vi "Allan-Variance_Algorithm.VI"(1 "tau":dbl, 2 "Input Array":dbl[](array[numeric])) -> (0 "Allan-Varianz (tau)":dbl)   [LabVIEW 2020]
uses:
  <vilib>/Analysis/baseanly.llb/Mean (DBL).vi
  <vilib>/Analysis/NI_AALBase.lvlib
panel:
  out "[y_mean(k+1) - y_mean(k)]**2":dbl[](array[numeric]) format="%_3f"
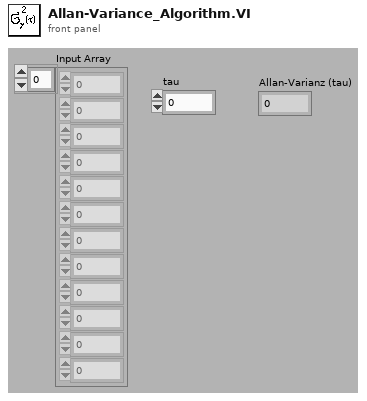
[diagram p1: front panel]
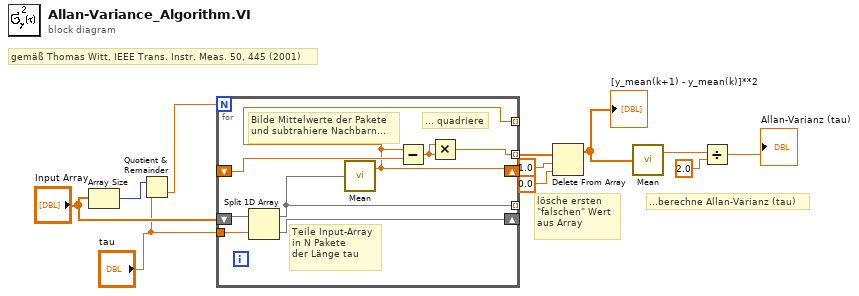
[diagram p0: block diagram]
diagram:
  # "gemäß Thomas Witt, IEEE Trans. Instr. Meas. 50, 445 (2001)"
  # "lösche ersten\n\"falschen\" Wert\naus Array"
  # "...berechne Allan-Varianz (tau)"
  n1 = Array Size(array="Input Array") -> (size(s)=w11:i32)
  n2 = Quotient & Remainder(x=w11, y="tau") -> (floor(x/y)=w8:dbl)  [unwired: 1 out]
  n3 = for {
    N: w8 -> [_]
    shift-right: [w17] -> _
    shift-left: "Input Array" -> [w18]
    tunnel: "tau" -> [w19]
    tunnel: [w16] -> _ mode=indexing
    shift-right: [w14] -> _
    shift-left: _ -> [w15]
    tunnel: [w12] -> w6 mode=indexing
    tunnel: [w14] -> _ mode=indexing
    # "... quadriere"
    # "Bilde Mittelwerte der Pakete\nund subtrahiere Nachbarn..."
    # "Teile Input-Array\nin N Pakete\nder Länge tau"
    n4 = Split 1D Array(array=w18, index=w19) -> (first subarray=w16:dbl[], second subarray=w17:dbl[])
    n5 = call-poly <vilib>:"Mean.vi"("X"=w16) -> ("mean"=w14:dbl)  [unwired: 1 out]
    n6 = Subtract(x=w14, y=w15) -> (x-y=w13:dbl)
    n7 = Multiply(x=w13, y=w13) -> (x*y=w12:dbl)
  }
  n8 = Delete From Array(array=w6, length=1.0 ("mean"), index=0.0 ("mean")) -> (array with subset deleted=w4:dbl[])  [unwired: 1 out]
  "[y_mean(k+1) - y_mean(k)]**2" <- w4
  n9 = call-poly <vilib>:"Mean.vi"("X"=w4) -> ("mean"=w3:dbl)  [unwired: 1 out]
  n10 = Divide(x=w3, y=2.0) -> (x/y=→"Allan-Varianz (tau)":dbl)
